vi "LVClass_CameraSet WriteFile CameraParametersSetup.vi"(0 "CameraSet in":refnum<class "CameraSet.lvclass">, 11 "error in (no error)":errorcluster) -> (4 "CameraSet out":refnum<class "CameraSet.lvclass">, 15 "error out":errorcluster)   [LabVIEW 2020, in "CameraSet.lvclass"]
uses:
  CameraSet.lvclass
  CameraSet.lvclass/CameraSet.ctl
  <vilib>/Utility/xml.llb/Write to XML File(string).vi
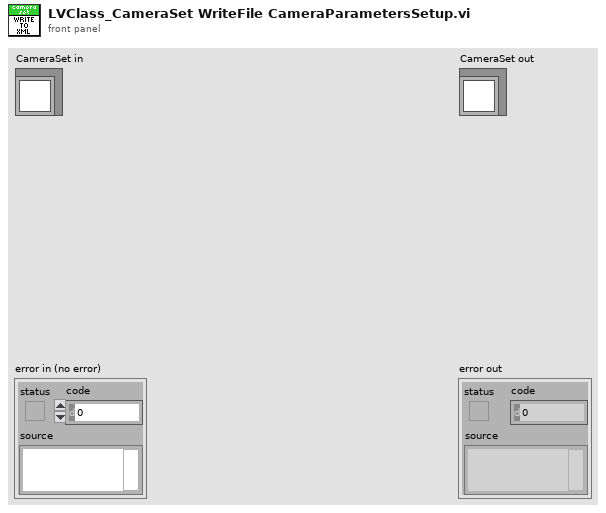
[diagram p1: front panel]
types:
  T1 = typedef "CameraParametersSetup.ctl" = cluster{"Name":string, "Type":T2, "Value":dbl, "BooleanValue":bool, "StringValue":string, "ConnectionParameter":bool}
  T2 = typedef "CameraParameters_Type.ctl" = enum16{"Integer", "Real", "String", "Boolean"}
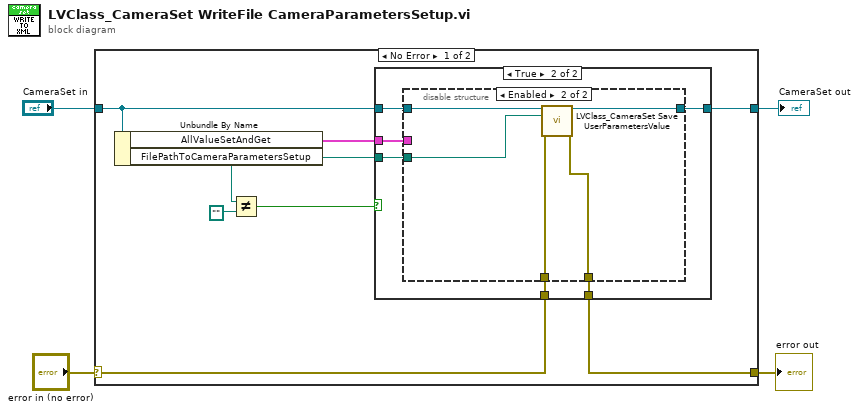
[diagram p0: block diagram]
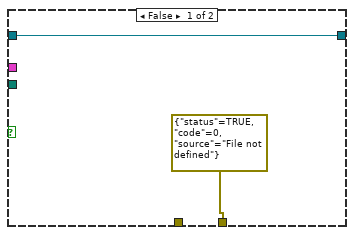
[diagram p2: hidden frame]
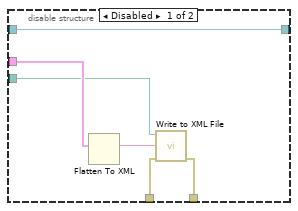
[diagram p3: hidden frame]
diagram:
  n1 = case shown="No Error" "error in (no error)" {
    selector: "error in (no error)" -> [w11 w33]
    tunnel: [w10 w33] -> w3
    tunnel: [w6 w32] -> w1
    tunnel: "CameraSet in" -> [w5 w32]
    frame No Error {
      n2 = Unbundle By Name(w5) -> ("AllValueSetAndGet"=w12:T1[], "FilePathToCameraParametersSetup"=w7:path)
      n3 = Not Equal?(x=w7, y=path "") -> (x != y?=w8:bool)
      n4 = case shown="True" w8 {
        tunnel: w12 -> [_ w20]
        tunnel: w7 -> [_ w19]
        tunnel: w11 -> [_ w18]
        tunnel: [errorcluster {"status"=TRUE, "code"=0, "source"="File not defined"} ("error out") w17] -> w10
        tunnel: [w13 w16] -> w6
        tunnel: w5 -> [w13 w15]
        frame False {
        }
        frame True {
          n5 = disable-structure shown="Enabled" {
            disable-tunnel: w20 -> [w26 _]
            disable-tunnel: w19 -> [w24 w30]
            disable-tunnel: w18 -> [w23 w28]
            disable-tunnel: [w22 w27] -> w17
            disable-tunnel: w15 -> [w21 w31]
            disable-tunnel: [w21 w29] -> w16
            frame Disabled {
              n6 = Flatten To XML(6:w26) -> (2:w25:string)
              n7 = call-poly <vilib>:"Write to XML File.vi"("error in (no error)"=w23, "XML Input"=w25, "XML File Path"=w24) -> ("error out"=w22:errorcluster)  [unwired: 6 in, 2 out]
            }
            frame Enabled {
              n8 = call "LVClass_CameraSet Save UserParametersValue.vi"("CameraSet.lvclass"=w31, "ParametersValue file path"=w30, "error in (no error)"=w28) -> ("CameraSet.lvclass"=w29:refnum<class "CameraSet.lvclass">, "error out"=w27:errorcluster)  [unwired: 11 in]
            }
          }
        }
      }
    }
    frame Error {
    }
  }
  "error out" <- w3
  "CameraSet out" <- w1
